vi "InsertCoin.vi"(8 "error in (no error)":errorcluster, 11 "State in":refnum<class "State.lvclass">) -> (0 "error out":errorcluster, 1 "NextState":T1=enum."有硬幣", 2 "ProcessMessage":string, 3 "State out":refnum<class "State.lvclass">)   [LabVIEW 2013, in "State.lvclass"]
uses:
  State.lvclass
  StateMark.ctl
panel:
  # "投入硬幣動作"
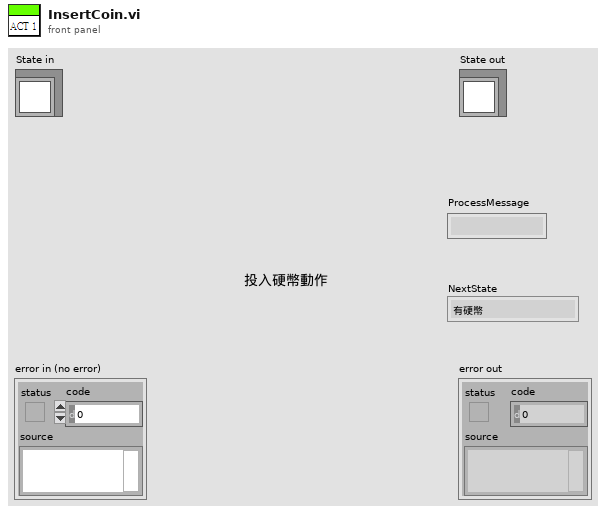
[diagram p1: front panel]
types:
  T1 = typedef "StateMark.ctl" = enum16{"沒有硬幣", "有硬幣", "賣出糖果", "糖果賣完", "NoChange"}
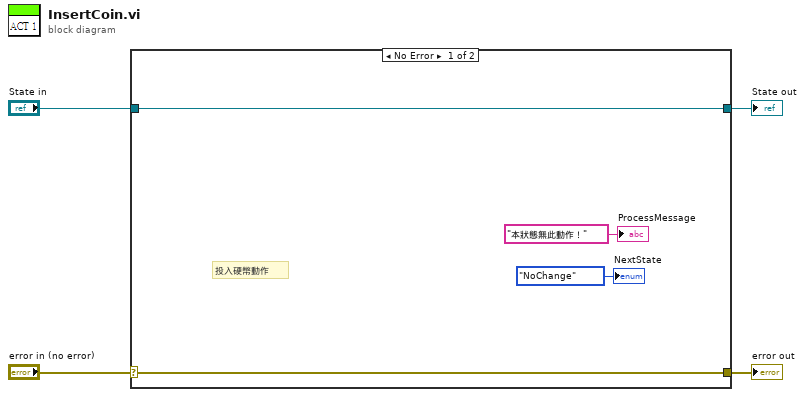
[diagram p0: block diagram]
diagram:
  n1 = case shown="No Error" "error in (no error)" {
    selector: "error in (no error)" -> [w8 w10]
    tunnel: [w8 w10] -> w3
    tunnel: [w7 w9] -> w1
    tunnel: "State in" -> [w7 w9]
    frame No Error {
      # "投入硬幣動作"
      "ProcessMessage" <- "本狀態無此動作！" ("ProcessMessage")
      "NextState" <- StateMark."NoChange" ("NextState")
    }
    frame Error {
    }
  }
  "error out" <- w3
  "State out" <- w1
